vi "IsImplemented.vi"(2 "error in (no error)":errorcluster, 3 "Feature Name":string, 4 "IGxDevice":refnum<k24>) -> (0 "error out":errorcluster, 1 "IsImplement":bool)   [LabVIEW 2013, in "GxLVlib.lvlib"]
uses:
  GxLVlib.lvlib
  C:/Program Files/Daheng Imaging/GalaxySDK/Samples/LabVIEW SDK/x86/GxLVLib/dll/GxIAPINET.dll
  dll/GxIAPINET.dll
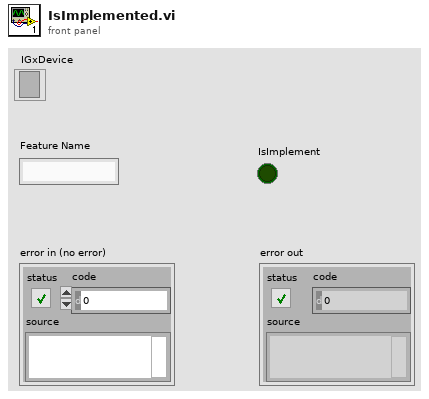
[diagram p1: front panel]
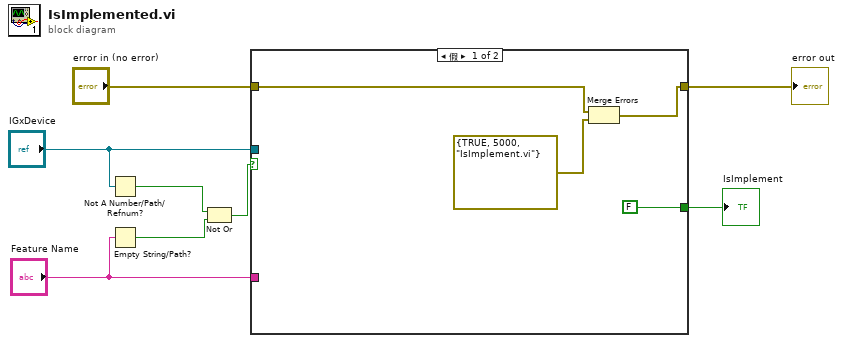
[diagram p0: block diagram]
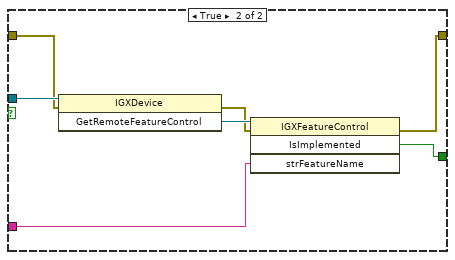
[diagram p2: hidden frame]
diagram:
  n1 = Not A Number/Path/Refnum?(number/path/refnum="IGxDevice") -> (NaN/Path/Refnum?=w8:bool)
  n2 = Empty String/Path?(string/path="Feature Name") -> (empty?=w7:bool)
  n3 = Not Or(1:w7, 2:w8) -> (0:w6:bool)
  n4 = case shown="假" w6 {
    tunnel: "error in (no error)" -> [w10 w18]
    tunnel: [w9 w13] -> w4
    tunnel: [FALSE w15] -> w3
    tunnel: "IGxDevice" -> [_ w19]
    tunnel: "Feature Name" -> [_ w16]
    frame False {
      n5 = Merge Errors(w10, errorcluster {TRUE, 5000, "IsImplement.vi"}) -> (w9:errorcluster)
    }
    frame True {
      n6 = invoke class="IGXDevice" method="GetRemoteFeatureControl"(reference=w19, error in=w18) -> (error out=w14:errorcluster, "GetRemoteFeatureControl"=w17:refnum<k24>)  [unwired: 1 in, 1 out]
      n7 = invoke class="IGXFeatureControl" method="IsImplemented"(reference=w17, error in=w14, "strFeatureName"=w16) -> (error out=w13:errorcluster, "IsImplemented"=w15:bool)  [unwired: 1 in, 2 out]
    }
  }
  "IsImplement" <- w3
  "error out" <- w4
